vi "Set Producer Values.vi"(8 "error in":errorcluster, 9 "Producer Ch":T1[](array[typedef])=[{"Error.STS"=0, "OutputEnable.STS"=0, "ControlMode.STS"=0, "Voltage.AV"=0.0, "Current.AV"=0.0, "Power.AV"=0.0}], 10 "Producer Control":T2, 11 "Power Supply Cluster.lvclass in":refnum<class "Power Supply Cluster.lvclass">) -> (0 "error out":errorcluster, 3 "Power Supply Cluster.lvclass out":refnum<class "Power Supply Cluster.lvclass">)   [LabVIEW 2023, in "Power Supply Cluster.lvclass"]
uses:
  Power Supply Cluster.lvclass
  Producer Control.ctl
  Producer Ch.ctl
  Power Supply Cluster.lvclass/Power Supply Cluster.ctl
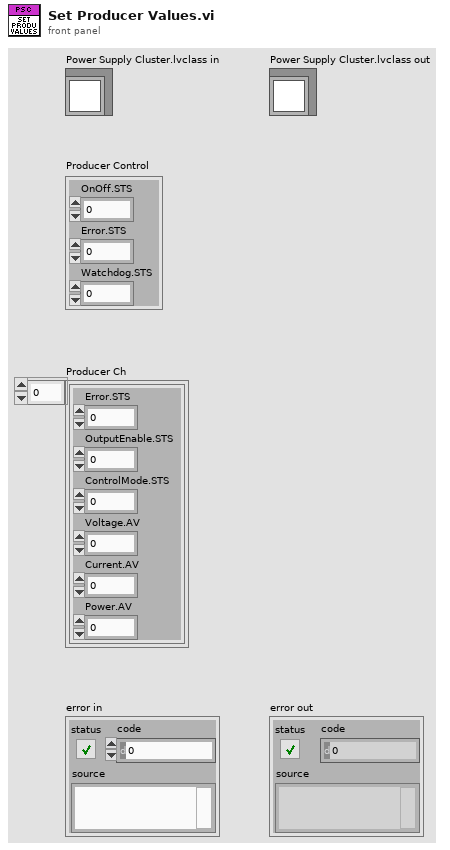
[diagram p1: front panel]
types:
  T1 = typedef "Power Supply Cluster.lvclass/Producer Ch.ctl" = cluster{"Error.STS":i32, "OutputEnable.STS":i32, "ControlMode.STS":u16, "Voltage.AV":dbl, "Current.AV":dbl, "Power.AV":dbl}
  T2 = typedef "Power Supply Cluster.lvclass/Producer Control.ctl" = cluster{"OnOff.STS":i32, "Error.STS":i32, "Watchdog.STS":i32}
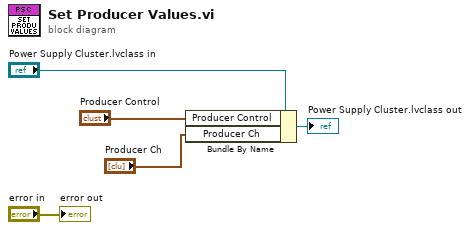
[diagram p0: block diagram]
diagram:
  n1 = Bundle By Name(cluster="Power Supply Cluster.lvclass in", "Producer Control"="Producer Control", "Producer Ch"="Producer Ch") -> (→"Power Supply Cluster.lvclass out":refnum<class "Power Supply Cluster.lvclass">)
  "error out" <- "error in"
